vi "Set_Number_of_UL_Antennas.vi"(8 "error in (no error)":errorcluster, 9 "No of UL antennas Value":i32=1, 10 "Cellular Technology":T1, 11 "Base Station":T2) -> (0 "error out":errorcluster, 3 "Output String":string)   [LabVIEW 2021]
uses:
  Controls/Base_Station_Emulator.ctl
  Controls/Cellular_Technology.ctl
  Controls/TCP_FGV.ctl
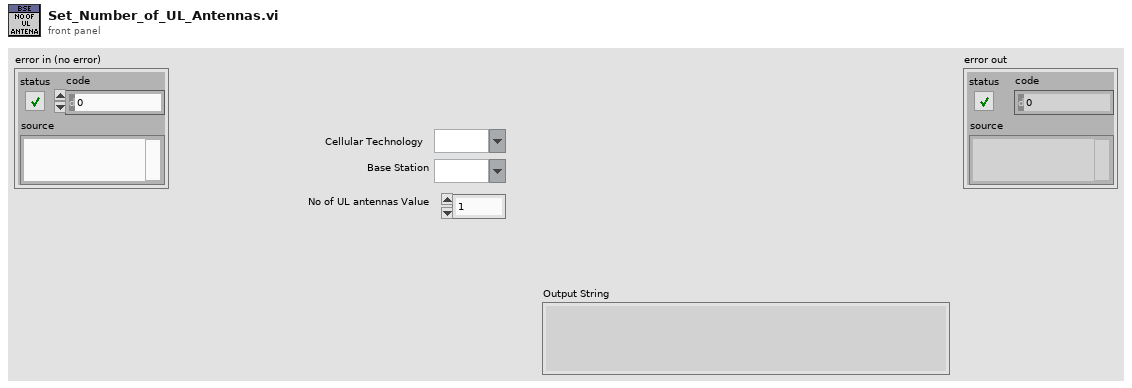
[diagram p1: front panel]
types:
  T1 = typedef "Cellular_Technology.ctl" = string
  T2 = typedef "Base_Station_Emulator.ctl" = string
  T3 = typedef "TCP_FGV.ctl" = enum16{"Open", "Read", "Write", "Close"}
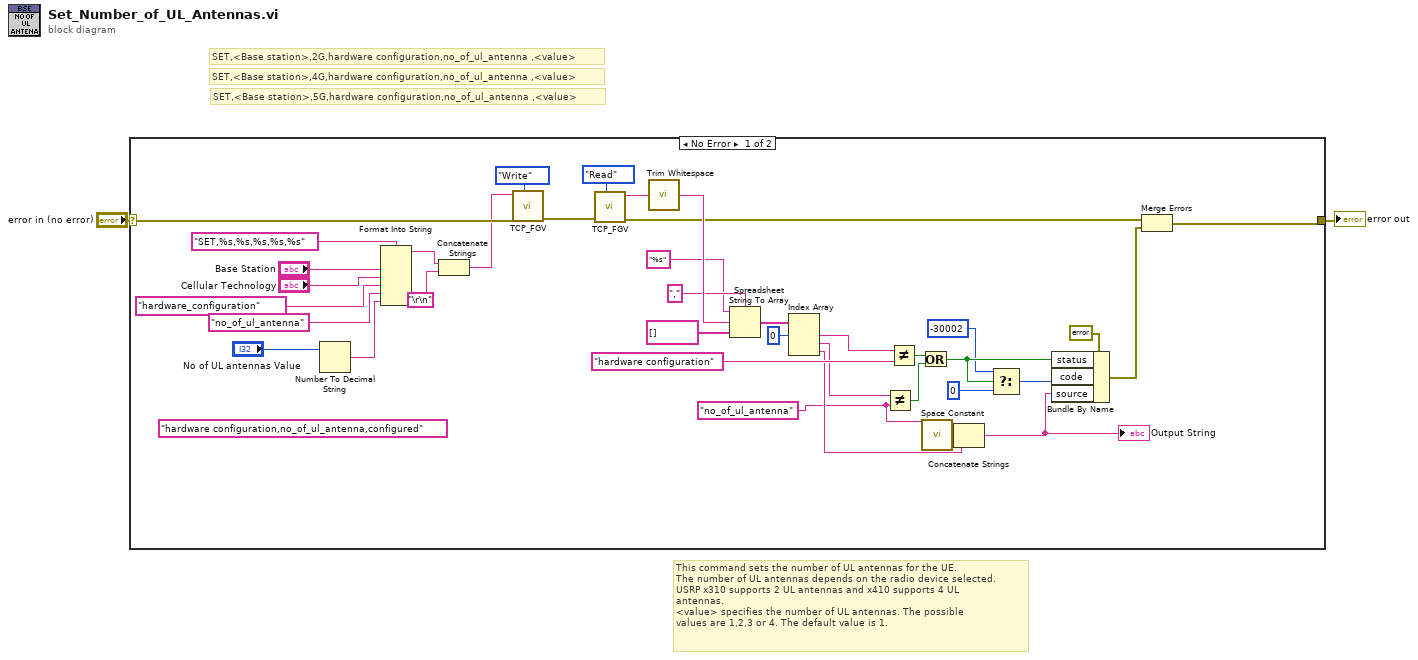
[diagram p0: block diagram]
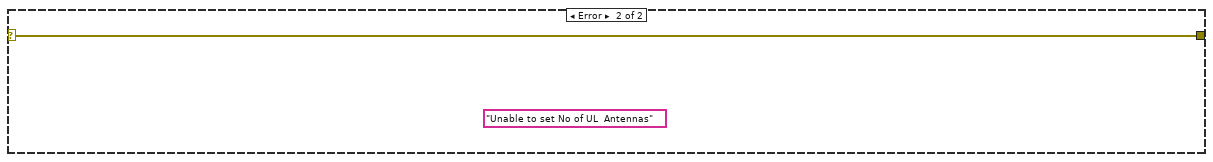
[diagram p2: hidden frame]
diagram:
  # "This command sets the number of UL antennas for the UE. \nThe number of UL antennas depends on the radio device selected. \nUSRP x310 supports 2 UL antennas and x410 supports 4 UL \nantennas.  \n<value> specifies the number of UL antennas. The possible \nvalues are 1,2,3 or 4. The default value is 1."
  # "SET,<Base station>,5G,hardware configuration,no_of_ul_antenna ,<value>"
  # "SET,<Base station>,4G,hardware configuration,no_of_ul_antenna ,<value>"
  # "SET,<Base station>,2G,hardware configuration,no_of_ul_antenna ,<value>"
  n1 = case shown="No Error" "error in (no error)" {
    selector: "error in (no error)" -> [w38 w41]
    tunnel: [w17 w41] -> w1
    frame No Error {
      (unwired) "hardware configuration,no_of_ul_antenna,configured" ("format string")
      w12 = "no_of_ul_antenna"
      n2 = Number To Decimal String(number="No of UL antennas Value") -> (decimal integer string=w4:string)  [unwired: 1 in]
      n3 = Format Into String(format string="SET,%s,%s,%s,%s,%s", "Base Station", "Cellular Technology", "hardware_configuration", "no_of_ul_antenna", w4) -> (resulting string=w7:string)  [unwired: 2 in, 1 out]
      n4 = Concatenate Strings(w7, "\r\n") -> (w6:string)
      n5 = call "TCP_FGV.vi"("Command"=w6, "error in (no error)"=w38, "Operation"=TCP_FGV."Write") -> ("error out"=w18:errorcluster)  [unwired: 6 in, 1 out]
      n6 = call "TCP_FGV.vi"("error in (no error)"=w18, "Operation"=TCP_FGV."Read") -> ("Data Out"=w15:string, "error out"=w20:errorcluster)  [unwired: 7 in]
      n7 = call <vilib>:"Trim Whitespace.vi"("string"=w15) -> ("trimmed string"=w31:string)  [unwired: 1 in]
      n8 = Spreadsheet String To Array(delimiter (Tab)=",", format string="%s", spreadsheet string=w31, array type (2D Dbl)=string[] []) -> (array=w35:string[])
      n9 = Index Array(array=w35, index #1=0 ("index")) -> (element #1=w34:string, element #2=w16:string, element #3=w13:string)  [unwired: 2 in]
      n10 = Not Equal?(x=w16, y=w12) -> (x != y?=w32:bool)
      n11 = Not Equal?(x=w34, y="hardware configuration" ("format string")) -> (x != y?=w33:bool)
      n12 = Or(x=w33, y=w32) -> (x .or. y?=w30:bool)
      n13 = call <vilib>:"Space Constant.vi"() -> ("String"=w14:string)
      n14 = Concatenate Strings(w12, w14, w13) -> (w11:string)
      "Output String" <- w11
      n15 = Select(t=-30002 ("code"), s=w30, f=0 ("code")) -> (s? t:f=w29:i32)
      n16 = Bundle By Name(cluster=errorcluster {"status"=FALSE, "code"=0, "source"=""} ("error constant"), "status"=w30, "code"=w29, "source"=w11) -> (w19:errorcluster)
      n17 = Merge Errors(w20, w19) -> (w17:errorcluster)
    }
    frame Error {
      (unwired) "Unable to set No of UL  Antennas" ("source")
    }
  }
  "error out" <- w1
